vi "Create Source Endpoints.vi"(8 "error in (no error)":errorcluster, 10 "Grouped Terminals":T2, 11 "Refs in":T1) -> (0 "error out":errorcluster, 3 "Refs":T1)   [LabVIEW 2020, in "FlexBlocks.lvlib"]
uses:
  FlexBlocks.lvlib
  Grouped Terminals.ctl
  Terminal Group.ctl
  Terminal Config.ctl
  Type Descriptor.ctl
  Terminal Direction.ctl
  Value Mode.ctl
  Special Terminal.ctl
  Terminal Mode.ctl
  Scripting Refs.ctl
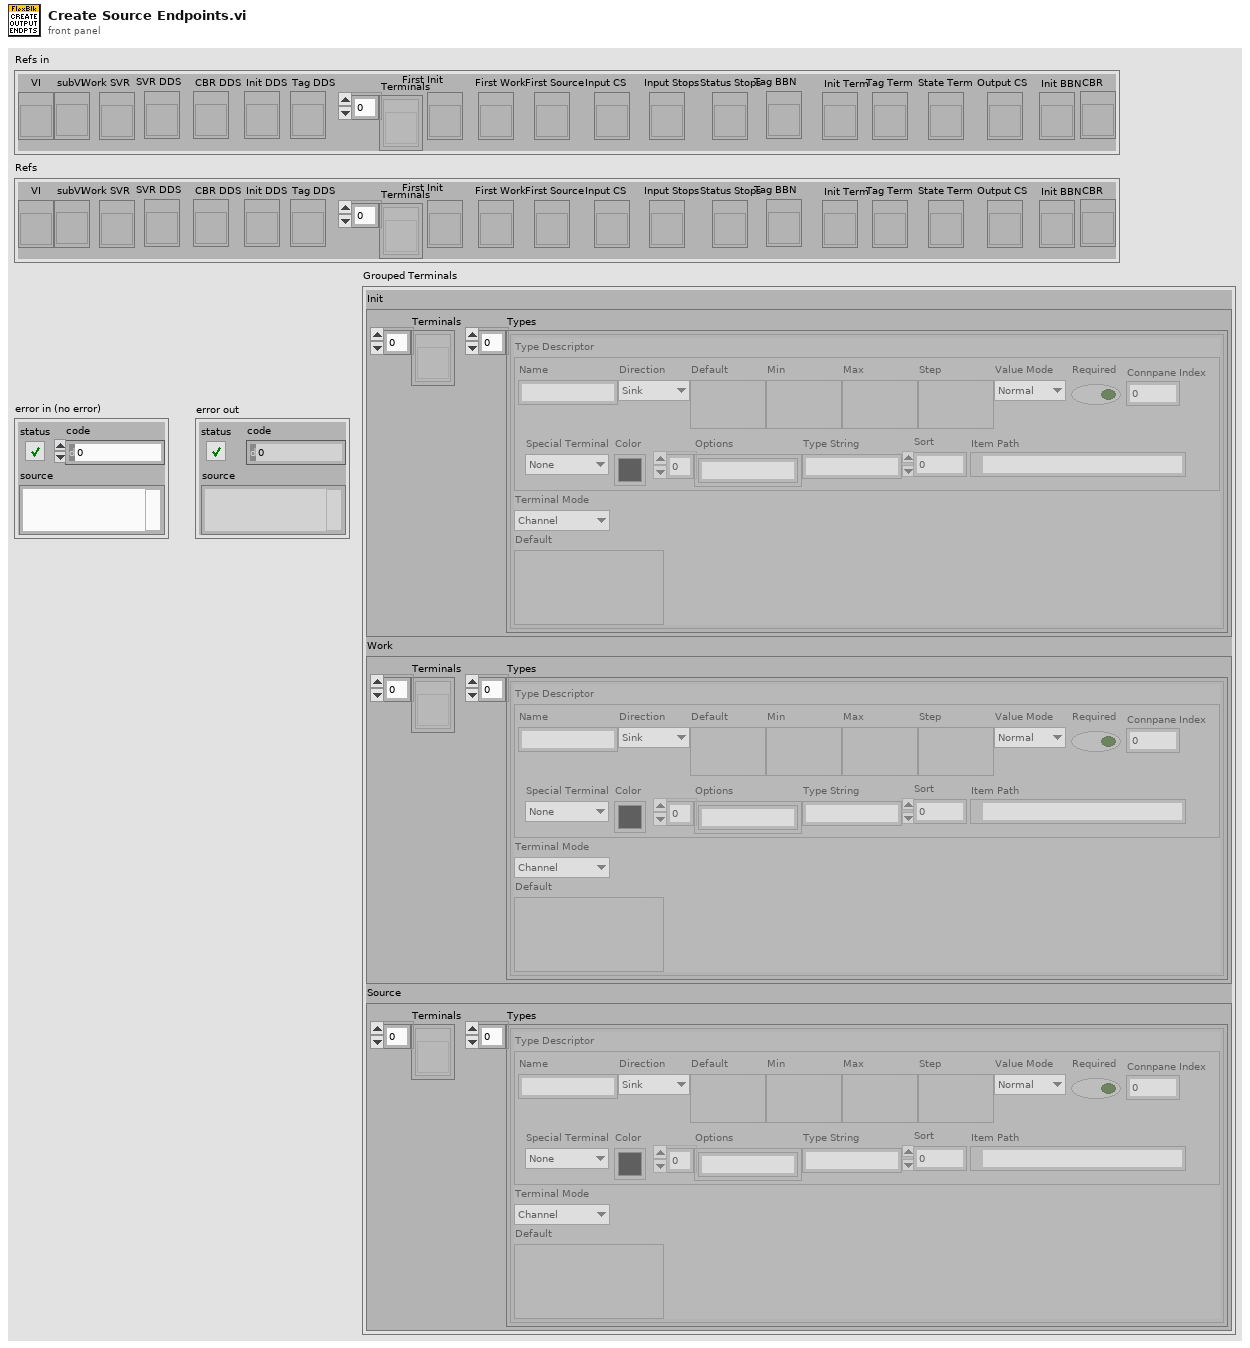
[diagram p1: front panel]
types:
  T1 = typedef "FlexBlocks.lvlib/Scripting Refs.ctl" = cluster{"VI":refnum<vi>, "subVI":refnum<vi>, "Work SVR":refnum<vi>, "SVR DDS":refnum<vi>, "CBR DDS":refnum<vi>, "Init DDS":refnum<vi>, "Tag DDS":refnum<vi>, "Terminals":refnum<vi>[], "First Init":refnum<vi>, "First Work":refnum<vi>, "First Source":refnum<vi>, "Input CS":refnum<vi>, "Input Stops":refnum<vi>, "Status Stops":refnum<vi>, "Tag BBN":refnum<vi>, "Init Term":refnum<vi>, "Tag Term":refnum<vi>, "State Term":refnum<vi>, "Output CS":refnum<vi>, "Init BBN":refnum<vi>, "CBR":refnum<vi>}
  T2 = typedef "FlexBlocks.lvlib/Grouped Terminals.ctl" = cluster{"Init":T3, "Work":T3, "Source":T3}
  T3 = typedef "FlexBlocks.lvlib/Terminal Group.ctl" = cluster{"Terminals":refnum<vi>[], "Types":T4[]}
  T4 = typedef "FlexBlocks.lvlib/Terminal Config.ctl" = cluster{"Type Descriptor":T5, "Terminal Mode":T9, "Default":variant}
  T5 = typedef "FlexBlocks.lvlib/Type Descriptor.ctl" = cluster{"Name":string, "Direction":T6, "Default":variant, "Min":variant, "Max":variant, "Step":variant, "Value Mode":T7, "Required":bool, "Connpane Index":i32, "Special Terminal":T8, "Color":u32, "Options":string[], "Type String":string, "Sort":i32, "Item Path":path}
  T6 = typedef "FlexBlocks.lvlib/Terminal Direction.ctl" = enum16{"Sink", "Source"}
  T7 = typedef "FlexBlocks.lvlib/Value Mode.ctl" = enum16{"Normal", "Range", "Select"}
  T8 = typedef "FlexBlocks.lvlib/Special Terminal.ctl" = enum16{"None", "Action", "Init", "Tag", "State in", "State out", "Error"}
  T9 = typedef "FlexBlocks.lvlib/Terminal Mode.ctl" = enum16{"Channel", "Config", "Value", "Control Ref"}
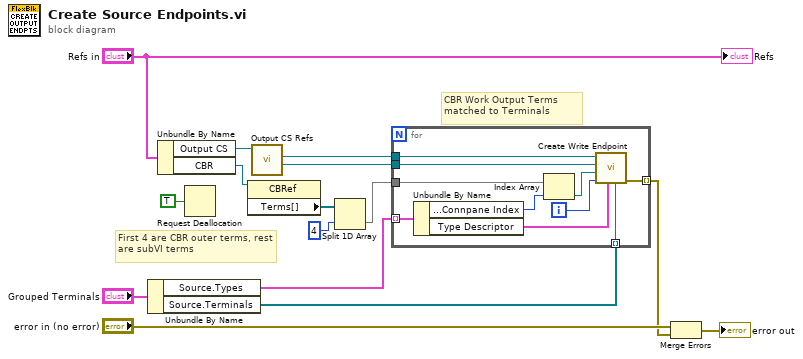
[diagram p0: block diagram]
diagram:
  # "CBR Work Output Terms matched to Terminals"
  # "First 4 are CBR outer terms, rest are subVI terms"
  n1 = Unbundle By Name("Grouped Terminals") -> ("Source.Types"=w11:T4[], "Source.Terminals"=w3:refnum<vi>[])
  n2 = Unbundle By Name("Refs in") -> ("Output CS"=w12:refnum<vi>, "CBR"=w10:refnum<vi>)
  n3 = Request Deallocation(TRUE ("flag")) -> ()
  n4 = property class="CBRef"(reference=w10) -> ("Terms[]"=w8:refnum<vi>[])  [unwired: 1 in, 2 out]
  n5 = call "Output CS Refs.vi"("Output CS in"=w12) -> ("Write Frame"=w6:refnum<vi>, "Close Term"=w5:refnum<vi>)  [unwired: 8 in, 1 out]
  n6 = Split 1D Array(array=w8, index=4) -> (second subarray=w7:refnum<vi>[])  [unwired: 1 out]
  n7 = for {
    tunnel: w11 -> [w20] mode=indexing
    tunnel: w7 -> [w25]
    tunnel: w6 -> [w23]
    tunnel: w5 -> [w22]
    tunnel: w3 -> [w17] mode=indexing
    tunnel: [w16] -> w1 mode=indexing
    i -> [w19]
    n8 = Unbundle By Name(w20) -> ("Type Descriptor.Connpane Index"=w24:i32, "Type Descriptor"=w18:T5)
    n9 = Index Array(array=w25, index=w24) -> (element=w21:refnum<vi>)
    n10 = call "Create Write Endpoint.vi"("Terminal"=w17, "Type"=w18, "Index"=w19, "CBR Terminal"=w21, "Close Tunnel"=w22, "Write Frame"=w23) -> ("error out"=w16:errorcluster)  [unwired: 5 in]
  }
  n11 = Merge Errors("error in (no error)", w1) -> (→"error out":errorcluster)
  "Refs" <- "Refs in"
